vi "Measure.vi"(6 "Init work":bool, 7 "Update period":dbl, 8 "error in (no error)":errorcluster, 9 "Last request":bool, 10 "Requester":string, 11 "Continuous Recorder in":refnum<class "Continuous Recorder.lvclass">) -> (0 "error out":errorcluster, 3 "Continuous Recorder out":refnum<class "Continuous Recorder.lvclass">)   [LabVIEW 2021, in "Continuous Recorder.lvclass"]
uses:
  Continuous Recorder.lvclass
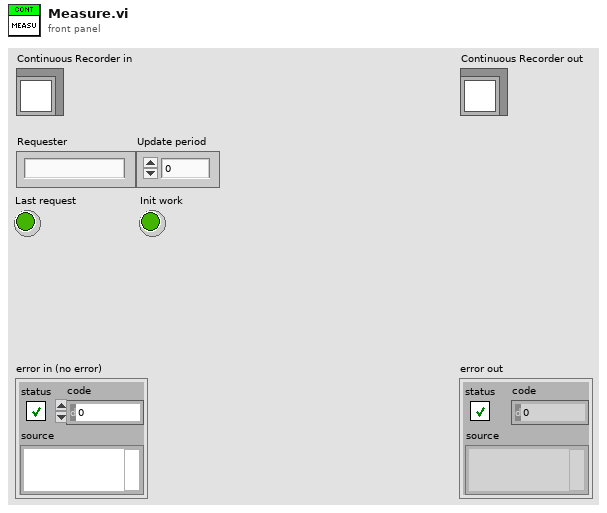
[diagram p1: front panel]
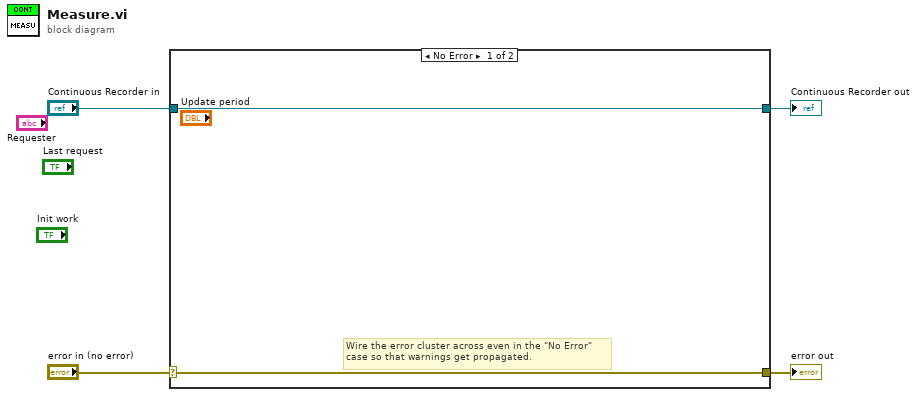
[diagram p0: block diagram]
diagram:
  n1 = case shown="No Error" "error in (no error)" {
    selector: "error in (no error)" -> [w5 w8]
    tunnel: [w5 w8] -> w3
    tunnel: [w6 w7] -> w1
    tunnel: "Continuous Recorder in" -> [w6 w7]
    frame No Error {
      # "Wire the error cluster across even in the \"No Error\"\ncase so that warnings get propagated."
    }
    frame Error {
    }
  }
  "error out" <- w3
  "Continuous Recorder out" <- w1
